vi "heating_visu OPC.vi"(7 "name":string="HT1", 9 "stop":bool, 10 "connect (T)":bool=TRUE) -> (0 "error out":errorcluster, 5 "This VI":refnum<vi>)   [LabVIEW 2019]
uses:
  ctl/Z_OnSwitch/Z_OnSwitch.xctl
  ctl/Z_ind_heating.ctl
  ctl/Z_Hswitch/Z_Hswitch.xctl
  ctl/YQ/YQ.xctl
  ctl/Y_SP/Y_SP.xctl
  ctl/Y_source.ctl
  ctl/Y_state.ctl
  ctl/Z_State.ctl
  ctl/ZM_State.ctl
  ctl/ZY_state_OPC.ctl
  ctl/ZY_state.ctl
  ctl/Z.ctl
  ctl/Y.ctl
  Inputs/Ctl/Parameter State.ctl
  Alarms/Ctl/ALR_Status.ctl
  <vilib>/OPCUA/controls/OPC UA StatusCode.ctl
  <vilib>/OPCUA/controls/Write Variant Request.ctl
  <vilib>/OPCUA/controls/NodeId.ctl
  <vilib>/OPCUA/controls/Write Status.ctl
  08a30d42-25e3-4a58-beca-1d562a75ea40.vi
  fbc51cc2-a17d-4d51-90ca-ef1d5e9adb43.vi
  3276b797-77fd-4487-96b2-8bfe15282525.vi
  81bac83f-5a8a-4521-9bb9-45d0222ee4c6.vi
  d9d9f7ca-8a59-4ad9-a7a4-c1f21956dc55.vi
  adc3267b-651c-4430-a21e-8a9f6f8285c6.vi
  45230f51-ed9d-4592-a49a-e0edfe92ddd1.vi
  Counter/Generator simplified.vi
  <vilib>/NI/AMC/Create Single Message.vi
  <vilib>/NI/AMC/Update Message Routing Info.vi
  <vilib>/NI/AMC/Read Termination Message.vi
  <vilib>/NI/AMC/Globals.vi
  <vilib>/NI/AMC/Send Message.vi
  Global stop.vi
  <vilib>/OPCUA/client/Multiple Read String.vi
  <vilib>/JDP Science/JSONtext/JSON text to Variant.vi
  <vilib>/OPCUA/client/Multiple Write Variant.vi
  Heating.lvlib
  <vilib>/OPCUA/NI OPC UA Client.lvlib
  OPC/OPC addons.lvlib
  Inputs/Inputs.lvlib
  <vilib>/NI/AMC/AMC.lvlib
  Alarms/Alarms.lvlib
panel:
  in  "Y_SP":cluster{dbl, dbl, dbl}(xcontrol)
  in  "message name":string="AI redefine"
  out "status":string
  in  "process":bool
  in  "state variables":cluster{"CurrentFile":path}
  in  "security policy":T1
  out "JSON string":string
  in  "JSON":string
  in  "Write controls":bool
  out "T stage":dbl format="%<%M:%S>t"
  in  "YQ":dbl(xcontrol)
  in  "ALRL1_reset":bool
  in  "ALRL2_reset":bool
  out "Z3 ind":T2
  out "PV":dbl(slide) caption="oC" scale=0.0..500.0 scale format="%#.1f"
  in  "Z_OnSwitch":bool(xcontrol)
  in  "Z_Hswitch":bool(xcontrol)
  in  "Y_Hswitch":bool(xcontrol)
  out "Z5 State":string
  out "Y output":dbl format="%.2f"
  # "PV"
  # "SP"
  # "Y"
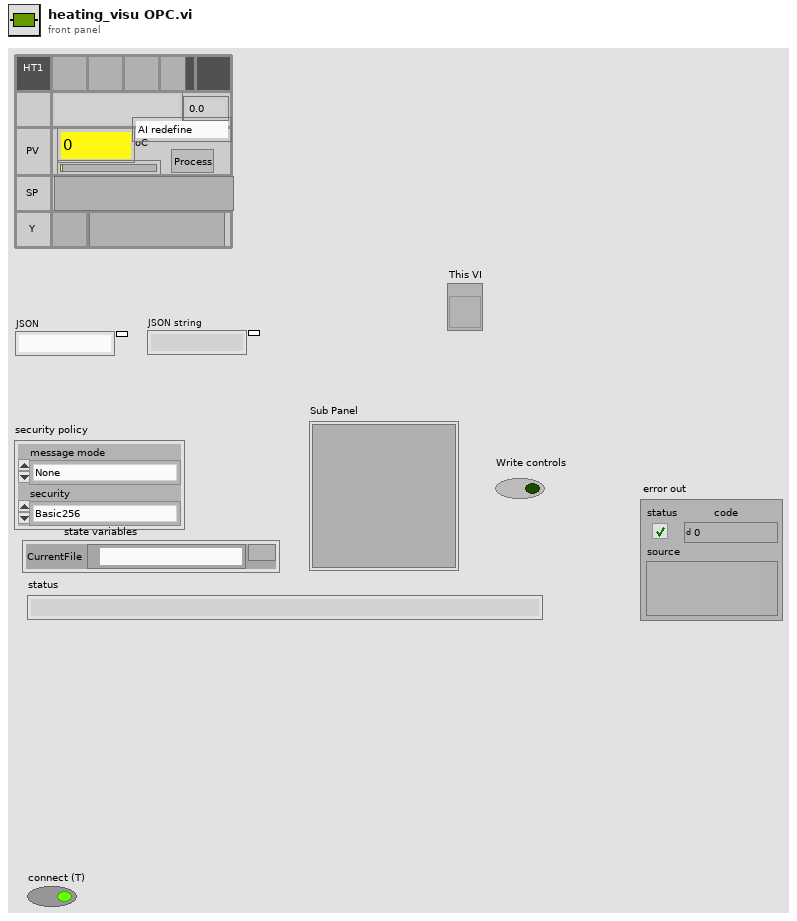
[diagram p1: front panel]
types:
  T1 = cluster{"message mode":enum16{"None", "Sign", "Sign and Encrypt"}, "security":enum16{"Basic256", "Basic128Rsa15"}}
  T2 = typedef "Heating.lvlib/Z_ind_heating.ctl" = u16
  T3 = typedef "AMC.lvlib/Message Queue.ctl" = refnum<queue>
  T4 = typedef "Write Variant Request.ctl" = cluster{"node ID":T5, "value":variant, "timestamp (current time)":timestamp, "node status":T6}
  T5 = typedef "NodeId.ctl" = string
  T6 = typedef "Write Status.ctl" = u32
  T7 = typedef "OPC UA Client Refnum.ctl" = refnum<k21>
  T8 = typedef "Subscription ID.ctl" = u32
  T9 = typedef "Heating.lvlib/Y_source.ctl" = enum8{"initialize", "local disabled", "local hand", "hand", "auto", "dist"}
  T10 = cluster{"connect":bool, "SP_Source":T9, "SP_Set":dbl, "SP":dbl}
  T11 = typedef "Heating.lvlib/Y_state.ctl" = enum8{"initialize", "alarm", "min", "stop", "hand", "auto", "max"}
  T12 = typedef "Heating.lvlib/Z_State.ctl" = enum8{"initialization", "alarm", "disabled", "not ready", "stop ready", "reserv", "switched off", "reserv2", "switched on", "check", "on min", "decrease out", "on", "increase out", "on max"}
  T13 = cluster{"connect":bool, "Z_Source":T9, "Z_State_heating":T12}
  T14 = typedef "Heating.lvlib/ZM_State.ctl" = enum8{"initialization", "stop", "start_cmd", "contactor_on_cmd", "heating", "on", "stop_cmd", "power_down", "contactor_off_cmd", "cooling", "restart_delay"}
  T15 = typedef "Heating.lvlib/ZY_state_OPC.ctl" = cluster{"Z":cluster{"Z_Source":u8, "Z_SetState":u8, "Z_State":u8, "Z_State_T":u32, "ZM_State":u8, "ZM_State_T":u32, "ALR  L1":bool, "ALR  L2":bool, "HH_run":i32}, "Y":cluster{"Y_Source":u8, "Y_SetState":u8, "SP_Set":dbl, "SP":dbl, "PV":dbl, "Y":dbl, "Y_State":cluster{"code":i32, "visible":bool, "color":u32}, "YB":bool}, "ALR_Status":cluster{"status":bool, "code":i32, "level":i32}[]}
  T16 = cluster{"Z_HSw":u32, "Z_HSetState":u32, "Y_HSw":u32, "Y_HSetState":u32, "SP":dbl, "Y_H":dbl, "Reset_ALR":bool}
  T17 = typedef "Heating.lvlib/ZY_state.ctl" = cluster{"Z":T18, "Y":T19, "ALR_Status":T21[]}
  T18 = typedef "Heating.lvlib/Z.ctl" = cluster{"Z_Source":T9, "Z_SetState":T12, "Z_State":T12, "Z_State_T":u32, "ZM_State":T14, "ZM_State_T":u32, "ALR  L1":bool, "ALR  L2":bool, "HH_run":i32}
  T19 = typedef "Heating.lvlib/Y.ctl" = cluster{"Y_Source":T9, "Y_SetState":T11, "SP_Set":dbl, "SP":dbl, "PV":dbl, "Y":dbl, "Y_State":T20, "YB":bool}
  T20 = typedef "Inputs.lvlib/Parameter State.ctl" = cluster{"code":i32, "visible":bool, "color":u32, "source":string}
  T21 = typedef "Alarms.lvlib/ALR_Status.ctl" = cluster{"status":bool, "code":i32, "level":i32, "source":string}
  T22 = typedef "OPC UA StatusCode.ctl" = u32
  T23 = enum32{"Invalid Status", "Unconnected", "Active", "Idle", "Error", "Connecting"}
  T24 = cluster{"node ID":T5, "value ":string, "timestamp":timestamp, "status":T22}[]
  T25 = typedef "LVDataSocketStatusTypeDef.ctl" = cluster{"Code":enum32{"Invalid Status", "Unconnected", "Active", "Idle", "Error", "Connecting"}, "Text":string}
  T26 = cluster{"node ID":T5, "value ":string, "timestamp":timestamp, "status":T22}
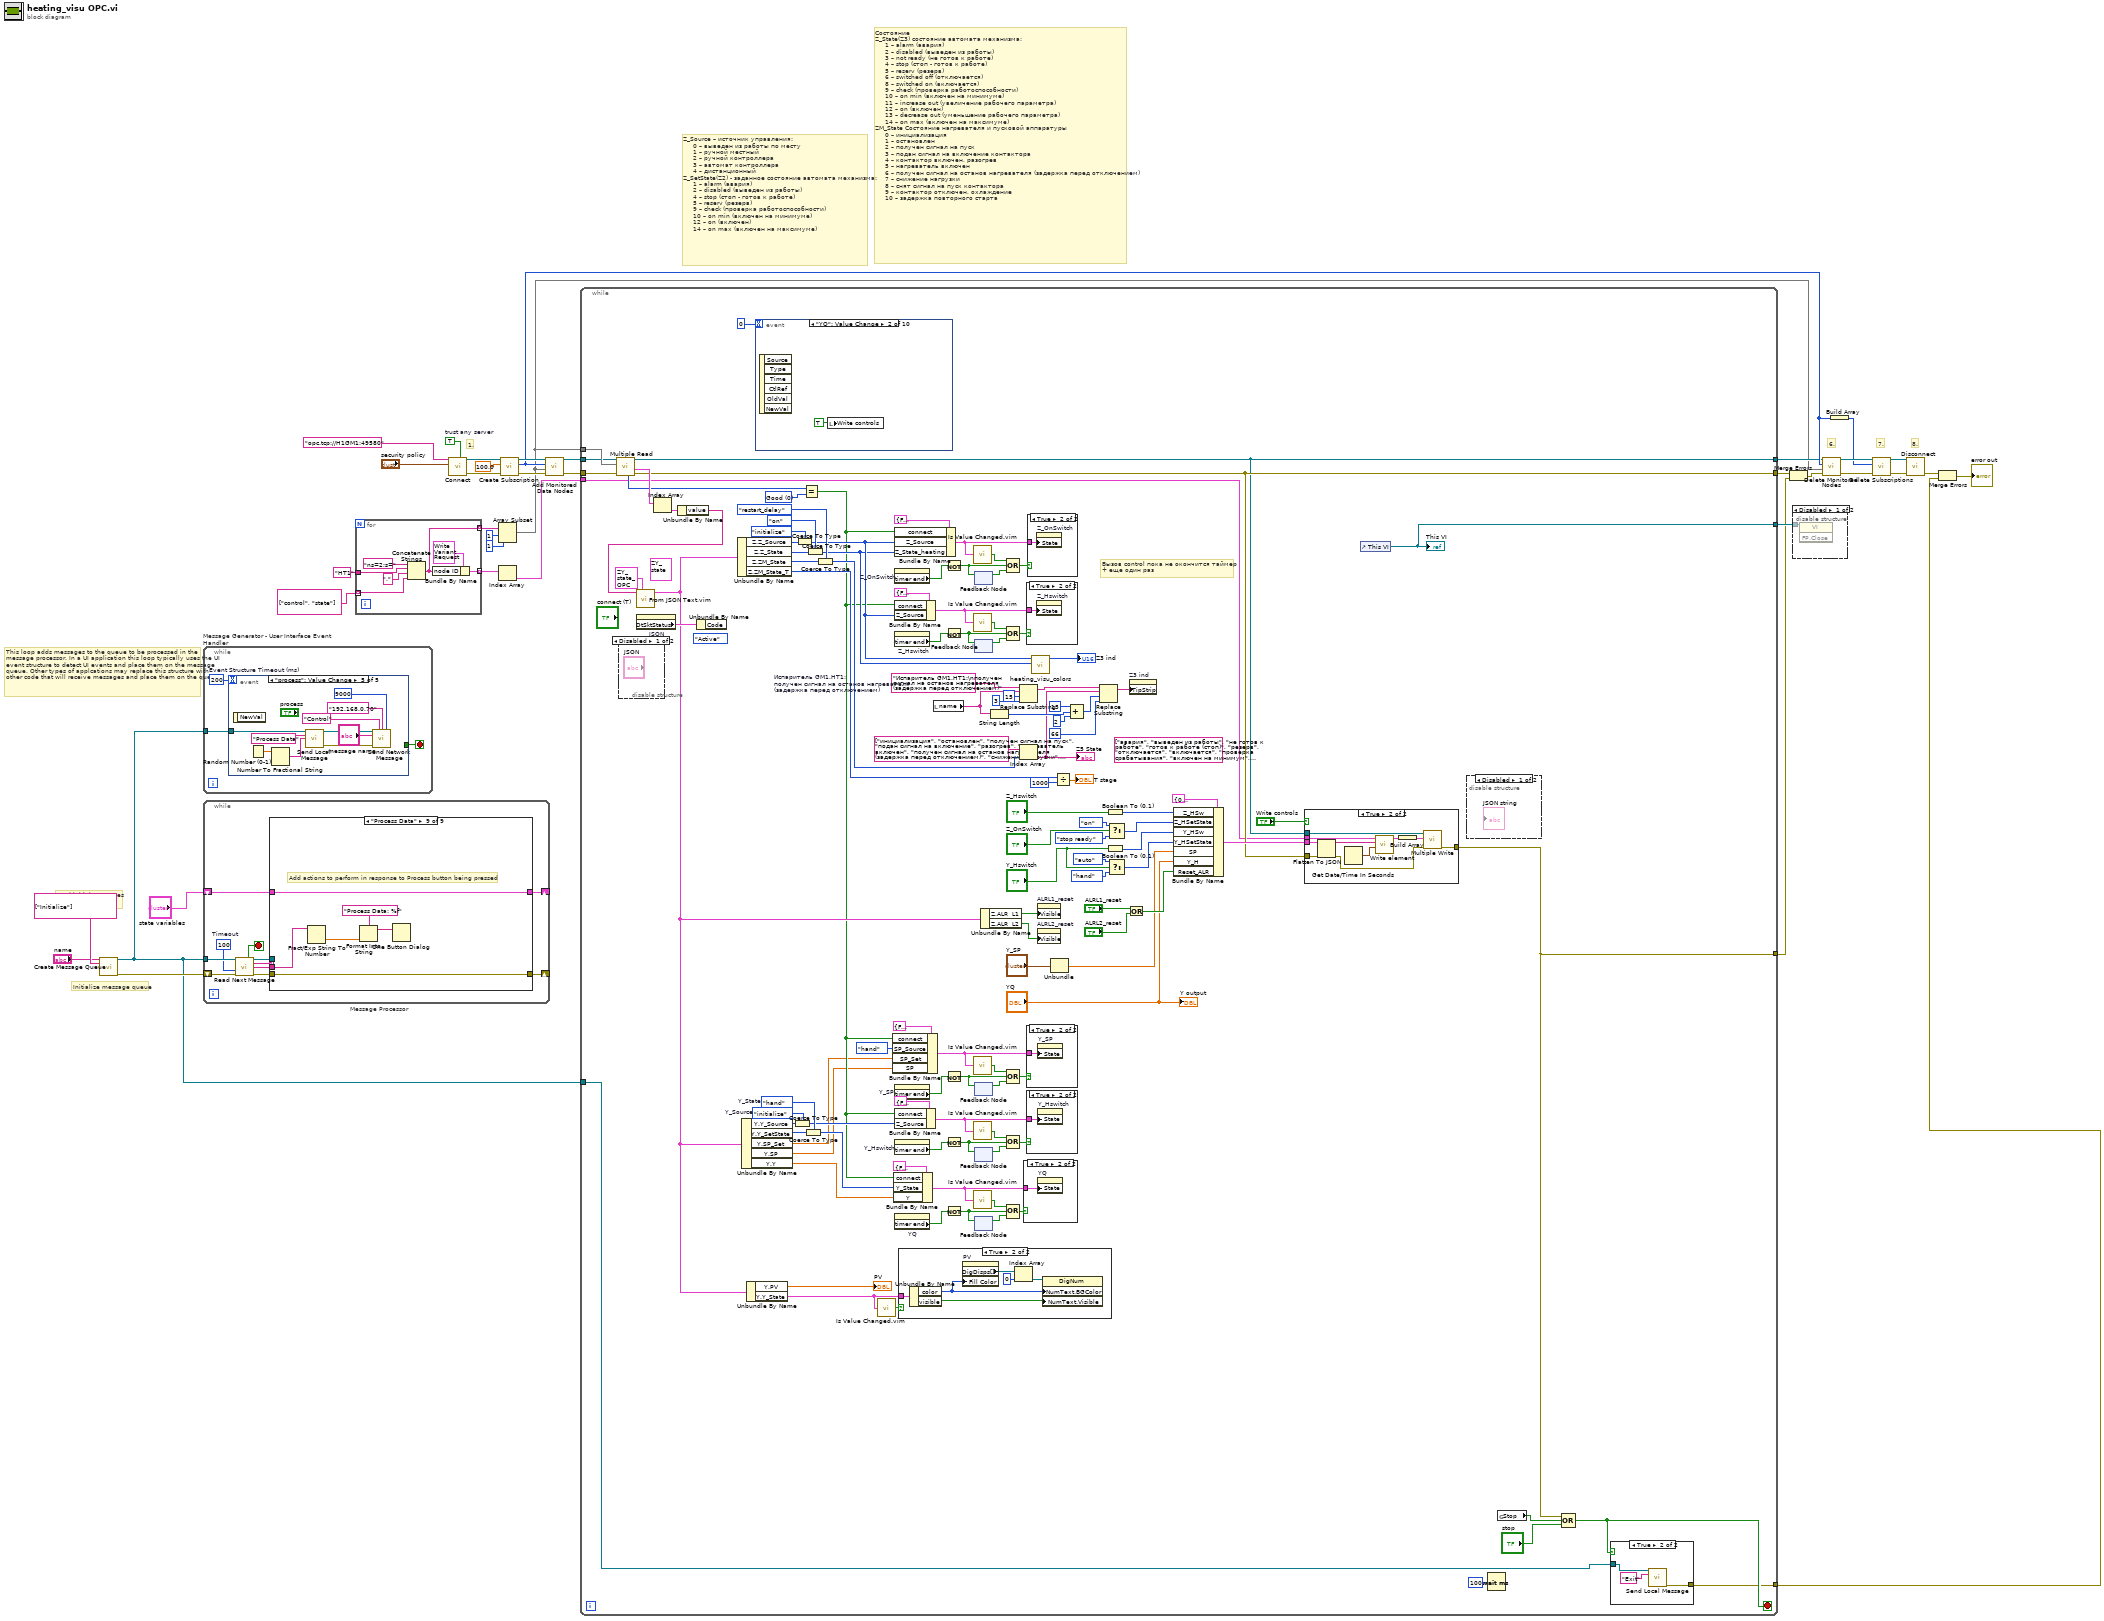
[diagram p0: block diagram]
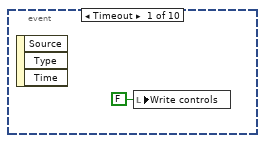
[diagram p9: hidden frame]
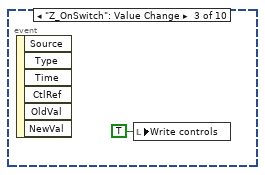
[diagram p10: hidden frame]
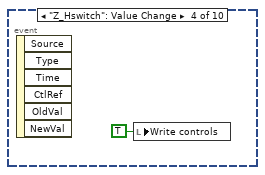
[diagram p11: hidden frame]
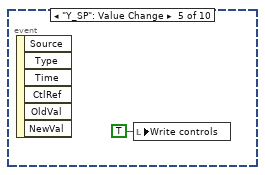
[diagram p12: hidden frame]
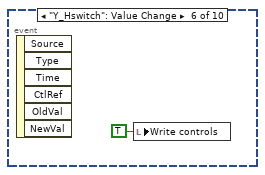
[diagram p13: hidden frame]
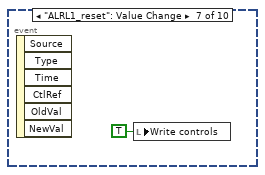
[diagram p14: hidden frame]
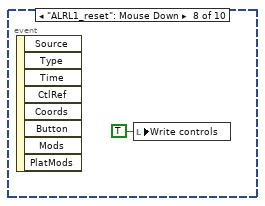
[diagram p15: hidden frame]
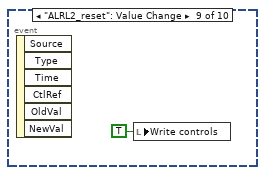
[diagram p16: hidden frame]
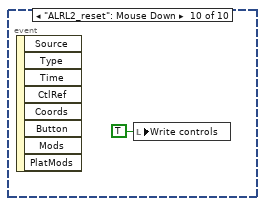
[diagram p17: hidden frame]
diagram:
  w30 = TRUE  # trust any server
  # "This loop adds messages to the queue to be processed in the message processor. In a UI application this loop typically uses the UI event structure to detect UI events and place them on the message queue. Other types of applcations may replace this structure with other code that will receive messages and place them on the queue."
  # "Initialize message queue"
  # "Load initial messages\non the queue"
  # "7."
  # "8."
  # "6."
  # "1."
  # "Состояние\nZ_State(Z3) состояние автомата механизма:\n     1 – alarm (авария)\n     2 – disabled (выведен из работы)\n     3 – not ready (не готов к работе)\n     4 – stop (стоп - готов к работе)\n     5 – reserv (резерв)\n     6 – switched off (отключается)\n     8 – switched on (включается)\n     9 – check (проверка работоспособности)\n     10 – on min (включен на минимуме)\n     11 – increase out (увеличение рабочего параметра)\n     12 – on (включен)\n     13 – decrease out (уменьшение рабочего параметра)\n     14 – on max (включен на максимуме)\nZM_State Состояние нагревателя и пусковой аппаратуры\n     0 – инициализация\n     1 – остановлен\n     2 – получен сигнал на пуск\n     3 – подан сигнал на включение контактора\n     4 – контактор включен, разогрев\n     5 – нагреватель включен\n     6 – получен сигнал на останов нагревателя (задержка перед отключением)\n     7 – снижение нагрузки\n     8 – снят сигнал на пуск контактора\n     9 – контактор отключен, охлаждение\n     10 – задержка повторного старта"
  # "Z_Source – источник управления:\n     0 – выведен из работы по месту\n     1 – ручной местный\n     2 – ручной контроллера\n     3 – автомат контроллера\n     4 – дистанционный\nZ_SetState(Z2) - заданное состояние автомата механизма:\n     1 – alarm (авария)\n     2 – disabled (выведен из работы)\n     4 – stop (стоп - готов к работе)\n     5 – reserv (резерв)\n     9 – check (проверка работоспособности)\n     10 – on min (включен на минимуме)\n     12 – on (включен)\n     14 – on max (включен на максимуме)"
  n1 = call <vilib>:"Create Message Queue.vi"("message queue name"="name", "initial message names"=string[] ["Initialize"]) -> ("message queue out"=w5:T3, "error out"=w7:errorcluster)  [unwired: 12 in]
  n2 = while "Message Generator - User Interface Event Handler" {
    tunnel: w5 -> [w38]
    stop <- w39 stop-if-true
    w40 = 200  # Event Structure Timeout (ms)
    n3 = event shown="[4] \"process\": Value Change" {
      selector: _ -> [_ _ _ _ _]
      dyn-events: _ -> [_ _ _ _ _]
      timeout: w40 -> [_ _ _ _ _]
      tunnel: [w41 w46 TRUE ("Discard?") _ _] -> w39
      tunnel: w38 -> [w42 w44 w47 w50 w61]
      event Timeout {
        # "Exit UI event handler loop if message queue\nis destroyed in the message processor"
        n4 = event-data() -> ()  [unwired: 2 out]
        n5 = call <vilib>:"Check Message Queue Status.vi"("message queue in"=w42) -> ("error out"=w43:errorcluster)  [unwired: 10 in, 4 out]
        n6 = Unbundle By Name(w43) -> ("status"=w41:bool)
        n7 = local write "stop"(w41) -> ()
      }
      event Panel Close? {
        w46 = TRUE ("Discard?")
        # "Intercepts the upper right close panel\noperation to allow a smooth shutdown\nas opposed to immediately killing the app."
        n8 = event-data() -> ()  [unwired: 2 out]
        n9 = call <vilib>:"Send Local Message.vi"("message queue in"=w44, "message name"="Exit") -> ()  [unwired: 11 in, 3 out]
        n10 = event-data("Discard?"=w46) -> ()  [unwired: 1 in, 1 out]
      }
      event "stop": Value Change {
        # "Exit the application\n>> Stop this message generator loop"
        n11 = event-data() -> ()  [unwired: 7 out]
        n12 = call <vilib>:"Send Local Message.vi"("message queue in"=w47, "message name"="Exit") -> ()  [unwired: 11 in, 3 out]
      }
      event Menu Selection (User) {
        # "Add run-time menu items to the message\nqueue. The message handler case names must match the menu ItemTag names."
        n13 = event-data() -> ("ItemTag"=w51:string)  [unwired: 1 out]
        n14 = call <vilib>:"Send Local Message.vi"("message queue in"=w50, "message name"=w51) -> ()  [unwired: 11 in, 3 out]
      }
      event "process": Value Change {
        n15 = event-data() -> ()  [unwired: 2 out]
        n16 = Random Number (0-1)() -> (number: 0 to 1=w58:dbl)
        n17 = Number To Fractional String(number=w58) -> (F-format string=w59:string)  [unwired: 3 out]
        n18 = call <vilib>:"Send Local Message.vi"("message queue in"=w61, "message name"="Process Data", "message value"=w59) -> ("message queue out"=w57:T3, "error out"=w53:errorcluster)  [unwired: 10 in, 1 out]
        n19 = call <vilib>:"Send Network Message.vi"("message queue in"=w57, "receiver process"="Control", "receiver host"="192.168.0.70", "receiver port (0)"=u16 9000, "message name"="message name", "error in"=w53) -> ()  [unwired: 7 in, 3 out]
      }
    }
  }
  n20 = while "Message Processor" {
    shift-left: w7 -> [w66]
    shift-right: [w70] -> _
    tunnel: w5 -> [w67]
    shift-left: "state variables" -> [w72]
    shift-right: [w71] -> _
    stop <- w69 stop-if-true
    w62 = 100  # Timeout
    n21 = call <vilib>:"Read Next Message.vi"("message queue in"=w67, "timeout (1 ms)"=w62, "error in"=w66) -> ("exit process?"=w69:bool, "message queue out"=w68:T3, "message name"=w64:string, "message value"=w63:string, "error out"=w65:errorcluster)  [unwired: 5 in, 3 out]
    n22 = case shown="\"Process Data\"" w64 {
      selector: w64 -> [_ _ w84 _ _ _ _ _ _]
      tunnel: [w74 w81 w86 w91 w93 w95 w100 w102 w107] -> w71
      tunnel: w72 -> [w74 w81 w86 w91 w93 w95 w100 w102 w107]
      tunnel: w68 -> [_ _ _ w89 _ _ w97 _ _]
      tunnel: w65 -> [w73 w80 w85 w87 w92 w94 w98 w101 w108]
      tunnel: [w73 w80 w85 errorcluster {"status"=FALSE, "code"=0, "source"=""} ("error out") w92 w94 w96 w101 w108] -> w70
      tunnel: w63 -> [_ _ _ _ _ _ _ _ w106]
      frame "---------- Framework Operations ----------" {
        # "Dummy case to add a seperator in the Case Structure menu"
      }
      frame "", "Idle" {
        # "Update the front panel"
        # "Idle Case - this case is called after a Timeout on the Get Next Message from Queue VI, if no new messages are present on the queue. This case can be used for housekeeping tasks such as updating the UI."
        n23 = Get Date/Time String(want seconds? (F)=TRUE) -> (date string=w79:string, time string=w78:string)  [unwired: 2 out]
        n24 = Concatenate Strings(w79, " " ("string"), w78) -> (→"status":string)
      }
      frame "Missing Message Handler", Default {
        # "Call this case if a message is received that is not handled \nby any other case. Typically this is a programming error\nas a result of a typo or unhandled message/missing message handler."
        n25 = Format Into String(format string="DevError: Missing message handler for '%s\" message." ("message"), w84) -> (resulting string=w82:string)  [unwired: 2 in, 1 out]
        n26 = One Button Dialog(message=w82) -> ()  [unwired: 2 out]
      }
      frame "Error" {
        # "Proceed to Exit - Remove this if it is\nnot appropriate for the General Error case"
        # "General Error Case - this case is called if an error is passed using the error cluster below. Typically most new errors should be handed in each individual case and not passed in the rror cluster. If necessary a custom error handler case should be added and called from other cases."
        n27 = call <vilib>:"Simple Error Handler.vi"("error in (no error)"=w87) -> ()  [unwired: 1 in, 8 out]
        n28 = call <vilib>:"Send Local Message.vi"("message queue in"=w89, "message name"="Exit") -> ()  [unwired: 11 in, 3 out]
      }
      frame "---------- Generic Operations ----------" {
        # "Dummy case to add a seperator in the Case Structure menu"
      }
      frame "Initialize" {
        # "Initialize the state variables and user interface"
      }
      frame "Exit" {
        # "Destroy message queue >> this will halt the UI event handler loop"
        # "Stop the VI\n>> Perform any cleanup tasks in this message case.\n>> Clear display before closing."
        n29 = call <vilib>:"Destroy Message Queue.vi"("message queue in"=w97, "error in"=w98) -> ("error out"=w96:errorcluster)  [unwired: 11 in, 2 out]
        n30 = local write "status"("" ("Status")) -> ()
      }
      frame "---------- Application Operations ----------" {
        # "Dummy case to add a seperator in the Case Structure menu"
      }
      frame "Process Data" {
        # "Add actions to perform in response to Process button being pressed"
        n31 = Fract/Exp String To Number(string=w106) -> (number=w105:dbl)  [unwired: 4 out]
        n32 = Format Into String(format string="Process Data: %f" ("message"), w105) -> (resulting string=w103:string)  [unwired: 2 in, 1 out]
        n33 = One Button Dialog(message=w103) -> ()  [unwired: 2 out]
      }
    }
  }
  n34 = for {
    tunnel: string[] ["control", "state"] -> [w109] mode=indexing
    tunnel: "HT1" ("Folder Name") -> [w115]
    tunnel: [w112] -> w19 mode=indexing
    tunnel: [w111] -> w15 mode=indexing
    n35 = Concatenate Strings("ns=2;s=" ("string"), w115, "." ("string"), w109) -> (w112:string)
    n36 = Bundle By Name(cluster=T4 {"node ID"="", "value"=variant, "timestamp (current time)"=timestamp(0 s since 1904-01-01), "node status"=0} ("request"), "node ID"=w112) -> (w111:T4)
  }
  n37 = call <vilib>:"Connect.vi"("trust any server (F)"=w30, "security policy"="security policy", "server endpoint URL"="opc.tcp://H1GM1:49580" ("server endpoint URL 2")) -> ("error out"=w33:errorcluster, "OPC UA client refnum out"=w34:T7)  [unwired: 6 in, 1 out]
  n38 = Array Subset(array=w19, index=1, length=1) -> (w9:string[])
  n39 = Index Array(array=w15) -> (element=w13:T4)  [unwired: 1 in]
  n40 = call <vilib>:"Create Subscription.vi"("error in (no error)"=w33, "publishing interval (1000 ms)"=100.0 ("update rate (1000 ms)"), "OPC UA client refnum in"=w34) -> ("error out"=w35:errorcluster, "subscription ID out"=w23:T8, "OPC UA client refnum out"=w36:T7)  [unwired: 4 in, 2 out]
  n41 = call <vilib>:"Add Monitored Data Nodes.vi"("error in (no error)"=w35, "node IDs"=w9, "subscription ID in"=w23, "OPC UA client refnum in"=w36) -> ("error out"=w16:errorcluster, "OPC UA client refnum out"=w17:T7)  [unwired: 4 in, 2 out]
  n42 = while {
    tunnel: [w198] -> w37
    tunnel: w17 -> [w187]
    tunnel: w16 -> [w194]
    tunnel: w13 -> [w186]
    tunnel: [w185] -> w12
    tunnel: [w187] -> w11
    tunnel: [w189] -> w10
    tunnel: w9 -> [w193]
    tunnel: w5 -> [w183]
    tunnel: [w182] -> w3
    stop <- w184 stop-if-true
    w170 = Y_state."hand"  # Y_State
    w171 = Y_source."initialize"  # Y_Source
    (unwired) T17 {"Z"={"Z_Source"=enum."initialize", "Z_SetState"=enum."initialization", "Z_State"=enum."initialization", "Z_State_T"=0, "ZM_State"=enum."initialization", "ZM_State_T"=0, "ALR  L1"=FALSE, "ALR  L2"=FALSE, "HH_run"=0}, "Y"={"Y_Source"=enum."initialize", "Y_SetState"=enum."initialize", "SP_Set"=0.0, "SP"=0.0, "PV"=0.0, "Y"=0.0, "Y_State"={"code"=0, "visible"=FALSE, "color"=0, "source"=""}, "YB"=FALSE}, "ALR_Status"=[]} ("HT1_state")
    w191 = T22 0 items=["Good"=0, "Good_SubscriptionTransferred"=2949120, "Good_CompletesAsynchronously"=3014656, "Good_Overload"=3080192, "Good_Clamped"=3145728, "Good_LocalOverride"=9830400, "Good_EntryInserted"=10616832, "Good_EntryReplaced"=10682368, "Good_NoData"=10813440, "Good_MoreData"=10878976, "Good_CommunicationEvent"=10944512, "Good_ShutdownEvent"=11010048, "Good_CallAgain"=11075584, "Good_NonCriticalTimeout"=11141120, "Good_ResultsMayBeIncomplete"=12189696, "Good_DataIgnored"=14221312, "Uncertain"=1073741824, "Uncertain_ReferenceOutOfServer"=1080819712, "Uncertain_NoCommunicationLastUsableValue"=1083113472, "Uncertain_LastUsableValue"=1083179008, "Uncertain_SubstituteValue"=1083244544, "Uncertain_InitialValue"=1083310080, "Uncertain_SensorNotAccurate"=1083375616, "Uncertain_EngineeringUnitsExceeded"=1083441152, "Uncertain_SubNormal"=1083506688, "Uncertain_DataSubNormal"=1084489728, "Uncertain_ReferenceNotDeleted"=1086062592, "Uncertain_NotAllNodesAvailable"=1086324736, "Bad"=2147483648, "Bad_UnexpectedError"=2147549184, "Bad_InternalError"=2147614720, "Bad_OutOfMemory"=2147680256, "Bad_ResourceUnavailable"=2147745792, "Bad_CommunicationError"=2147811328, "Bad_EncodingError"=2147876864, "Bad_DecodingError"=2147942400, "Bad_EncodingLimitsExceeded"=2148007936, "Bad_UnknownResponse"=2148073472, "Bad_Timeout"=2148139008, "Bad_ServiceUnsupported"=2148204544, "Bad_Shutdown"=2148270080, "Bad_ServerNotConnected"=2148335616, "Bad_ServerHalted"=2148401152, "Bad_NothingToDo"=2148466688, "Bad_TooManyOperations"=2148532224, "Bad_DataTypeIdUnknown"=2148597760, "Bad_CertificateInvalid"=2148663296, "Bad_SecurityChecksFailed"=2148728832, "Bad_CertificateTimeInvalid"=2148794368, "Bad_CertificateIssuerTimeInvalid"=2148859904, "Bad_CertificateHostNameInvalid"=2148925440, "Bad_CertificateUriInvalid"=2148990976, "Bad_CertificateUseNotAllowed"=2149056512, "Bad_CertificateIssuerUseNotAllowed"=2149122048, "Bad_CertificateUntrusted"=2149187584, "Bad_CertificateRevocationUnknown"=2149253120, "Bad_CertificateIssuerRevocationUnknown"=2149318656, "Bad_CertificateRevoked"=2149384192, "Bad_CertificateIssuerRevoked"=2149449728, "Bad_UserAccessDenied"=2149515264, "Bad_IdentityTokenInvalid"=2149580800, "Bad_IdentityTokenRejected"=2149646336, "Bad_SecureChannelIdInvalid"=2149711872, "Bad_InvalidTimestamp"=2149777408, "Bad_NonceInvalid"=2149842944, "Bad_SessionIdInvalid"=2149908480, "Bad_SessionClosed"=2149974016, "Bad_SessionNotActivated"=2150039552, "Bad_SubscriptionIdInvalid"=2150105088, "Bad_RequestHeaderInvalid"=2150236160, "Bad_TimestampsToReturnInvalid"=2150301696, "Bad_RequestCancelledByClient"=2150367232, "Bad_NoCommunication"=2150694912, "Bad_WaitingForInitialData"=2150760448, "Bad_NodeIdInvalid"=2150825984, "Bad_NodeIdUnknown"=2150891520, "Bad_AttributeIdInvalid"=2150957056, "Bad_IndexRangeInvalid"=2151022592, "Bad_IndexRangeNoData"=2151088128, "Bad_DataEncodingInvalid"=2151153664, "Bad_DataEncodingUnsupported"=2151219200, "Bad_NotReadable"=2151284736, "Bad_NotWritable"=2151350272, "Bad_OutOfRange"=2151415808, "Bad_NotSupported"=2151481344, "Bad_NotFound"=2151546880, "Bad_ObjectDeleted"=2151612416, "Bad_NotImplemented"=2151677952, "Bad_MonitoringModeInvalid"=2151743488, "Bad_MonitoredItemIdInvalid"=2151809024, "Bad_MonitoredItemFilterInvalid"=2151874560, "Bad_MonitoredItemFilterUnsupported"=2151940096, "Bad_FilterNotAllowed"=2152005632, "Bad_StructureMissing"=2152071168, "Bad_EventFilterInvalid"=2152136704, "Bad_ContentFilterInvalid"=2152202240, "Bad_FilterOperandInvalid"=2152267776, "Bad_ContinuationPointInvalid"=2152333312, "Bad_NoContinuationPoints"=2152398848, "Bad_ReferenceTypeIdInvalid"=2152464384, "Bad_BrowseDirectionInvalid"=2152529920, "Bad_NodeNotInView"=2152595456, "Bad_ServerUriInvalid"=2152660992, "Bad_ServerNameMissing"=2152726528, "Bad_DiscoveryUrlMissing"=2152792064, "Bad_SempahoreFileMissing"=2152857600, "Bad_RequestTypeInvalid"=2152923136, "Bad_SecurityModeRejected"=2152988672, "Bad_SecurityPolicyRejected"=2153054208, "Bad_TooManySessions"=2153119744, "Bad_UserSignatureInvalid"=2153185280, "Bad_ApplicationSignatureInvalid"=2153250816, "Bad_NoValidCertificates"=2153316352, "Bad_RequestCancelledByRequest"=2153381888, "Bad_ParentNodeIdInvalid"=2153447424, "Bad_ReferenceNotAllowed"=2153512960, "Bad_NodeIdRejected"=2153578496, "Bad_NodeIdExists"=2153644032, "Bad_NodeClassInvalid"=2153709568, "Bad_BrowseNameInvalid"=2153775104, "Bad_BrowseNameDuplicated"=2153840640, "Bad_NodeAttributesInvalid"=2153906176, "Bad_TypeDefinitionInvalid"=2153971712, "Bad_SourceNodeIdInvalid"=2154037248, "Bad_TargetNodeIdInvalid"=2154102784, "Bad_DuplicateReferenceNotAllowed"=2154168320, "Bad_InvalidSelfReference"=2154233856, "Bad_ReferenceLocalOnly"=2154299392, "Bad_NoDeleteRights"=2154364928, "Bad_ServerIndexInvalid"=2154430464, "Bad_ViewIdUnknown"=2154496000, "Bad_TooManyMatches"=2154627072, "Bad_QueryTooComplex"=2154692608, "Bad_NoMatch"=2154758144, "Bad_MaxAgeInvalid"=2154823680, "Bad_HistoryOperationInvalid"=2154889216, "Bad_HistoryOperationUnsupported"=2154954752, "Bad_WriteNotSupported"=2155020288, "Bad_TypeMismatch"=2155085824, "Bad_MethodInvalid"=2155151360, "Bad_ArgumentsMissing"=2155216896, "Bad_TooManySubscriptions"=2155282432, "Bad_TooManyPublishRequests"=2155347968, "Bad_NoSubscription"=2155413504, "Bad_SequenceNumberUnknown"=2155479040, "Bad_MessageNotAvailable"=2155544576, "Bad_InsufficientClientProfile"=2155610112, "Bad_TcpServerTooBusy"=2155675648, "Bad_TcpMessageTypeInvalid"=2155741184, "Bad_TcpSecureChannelUnknown"=2155806720, "Bad_TcpMessageTooLarge"=2155872256, "Bad_TcpNotEnoughResources"=2155937792, "Bad_TcpInternalError"=2156003328, "Bad_TcpEndpointUrlInvalid"=2156068864, "Bad_RequestInterrupted"=2156134400, "Bad_RequestTimeout"=2156199936, "Bad_SecureChannelClosed"=2156265472, "Bad_SecureChannelTokenUnknown"=2156331008, "Bad_SequenceNumberInvalid"=2156396544, "Bad_ConfigurationError"=2156462080, "Bad_NotConnected"=2156527616, "Bad_DeviceFailure"=2156593152, "Bad_SensorFailure"=2156658688, "Bad_OutOfService"=2156724224, "Bad_DeadbandFilterInvalid"=2156789760, "Bad_RefreshInProgress"=2157379584, "Bad_ConditionAlreadyDisabled"=2157445120, "Bad_ConditionDisabled"=2157510656, "Bad_EventIdUnknown"=2157576192, "Bad_NoData"=2157641728, "Bad_DataLost"=2157772800, "Bad_DataUnavailable"=2157838336, "Bad_EntryExists"=2157903872, "Bad_NoEntryExists"=2157969408, "Bad_TimestampNotSupported"=2158034944, "Bad_InvalidArgument"=2158690304, "Bad_ConnectionRejected"=2158755840, "Bad_Disconnect"=2158821376, "Bad_ConnectionClosed"=2158886912, "Bad_InvalidState"=2158952448, "Bad_EndOfStream"=2159017984, "Bad_NoDataAvailable"=2159083520, "Bad_WaitingForResponse"=2159149056, "Bad_OperationAbandoned"=2159214592, "Bad_ExpectedStreamToBlock"=2159280128, "Bad_WouldBlock"=2159345664, "Bad_SyntaxError"=2159411200, "Bad_MaxConnectionsReached"=2159476736, "Bad_RequestTooLarge"=2159542272, "Bad_ResponseTooLarge"=2159607808, "Bad_EventNotAcknowledgeable"=2159738880, "Bad_InvalidTimestampArgument"=2159869952, "Bad_ProtocolVersionUnsupported"=2159935488, "Bad_StateNotActive"=2160001024, "Bad_FilterOperatorInvalid"=2160132096, "Bad_FilterOperatorUnsupported"=2160197632, "Bad_FilterOperandCountMismatch"=2160263168, "Bad_FilterElementInvalid"=2160328704, "Bad_FilterLiteralInvalid"=2160394240, "Bad_IdentityChangeNotSupported"=2160459776, "Bad_NotTypeDefinition"=2160590848, "Bad_ViewTimestampInvalid"=2160656384, "Bad_ViewParameterMismatch"=2160721920, "Bad_ViewVersionInvalid"=2160787456, "Bad_ConditionAlreadyEnabled"=2160852992, "Bad_DialogNotActive"=2160918528, "Bad_DialogResponseInvalid"=2160984064, "Bad_ConditionBranchAlreadyAcked"=2161049600, "Bad_ConditionBranchAlreadyConfirmed"=2161115136, "Bad_ConditionAlreadyShelved"=2161180672, "Bad_ConditionNotShelved"=2161246208, "Bad_ShelvingTimeOutOfRange"=2161311744, "Bad_AggregateListMismatch"=2161377280, "Bad_AggregateNotSupported"=2161442816, "Bad_AggregateInvalidInputs"=2161508352, "Bad_BoundNotFound"=2161573888, "Bad_BoundNotSupported"=2161639424, "Bad_AggregateConfigurationRejected"=2161770496, "Bad_TooManyMonitoredItems"=2161836032] ("y")
    (unwired) T23."Active" ("Code")
    (unwired) string[] ["авария", "выведен из работы", "не готов к работе", "готов к работе (стоп)", "резерв", "отключается", "включается", "проверка срабатывания", "включен на минимум", "увеличение произв", "включен", "уменьшение произв", "включен на максимум"]
    w231 = "Испаритель GM1.HT1:\nполучен сигнал на останов нагревателя (задержка перед отключением)"  # Испаритель GM1.HT1: получен сигнал на останов нагревателя (задержка перед отключением)
    # "Вызов control пока не окончится таймер\n+ еще один раз"
    n43 = call-poly <vilib>:"Multiple Read.vi"("error in (no error)"=w194, "node IDs"=w193, "OPC UA client refnum in"=w187) -> ("error out"=w189:errorcluster, "results"=w196:T24, "service status"=w192:T22)  [unwired: 5 in, 1 out]
    n44 = disable-structure shown="Disabled" {
      frame Disabled {
      }
      frame Enabled {
      }
    }
    n45 = property on="JSON" class="Str"() -> ("DtSktStatus"=w199:T25)  [unwired: 2 in, 2 out]
    n46 = Index Array(array=w196) -> (element=w195:T26)  [unwired: 1 in]
    n47 = Unbundle By Name(w195) -> ("value"=w188:string)
    n48 = call "From JSON Text.vim"("Data Type and Default Value"=T15 {"Z"={"Z_Source"=0, "Z_SetState"=0, "Z_State"=0, "Z_State_T"=0, "ZM_State"=0, "ZM_State_T"=0, "ALR  L1"=FALSE, "ALR  L2"=FALSE, "HH_run"=0}, "Y"={"Y_Source"=0, "Y_SetState"=0, "SP_Set"=0.0, "SP"=0.0, "PV"=0.0, "Y"=0.0, "Y_State"={"code"=0, "visible"=FALSE, "color"=0}, "YB"=FALSE}, "ALR_Status"=[]} ("ZY_State"), "JSON"=w188) -> ("Data out"=w134:T15)  [unwired: 8 in, 1 out]
    n49 = Unbundle By Name(w199) -> ()  [unwired: 1 out]
    n50 = Unbundle By Name(w134) -> ("Z.Z_Source"=w177:u8, "Z.Z_State"=w211:u8, "Z.ZM_State"=w206:u8, "Z.ZM_State_T"=w213:u32)
    n51 = Unbundle By Name(w134) -> ("Y.Y_Source"=w176:u8, "Y.Y_SetState"=w212:u8, "Y.SP_Set"=w120:dbl, "Y.SP"=w119:dbl, "Y.Y"=w130:dbl)
    n52 = Unbundle By Name(w134) -> ("Y.PV"=→"PV":dbl, "Y.Y_State"=w132:cluster{"code":i32, "visible":bool, "color":u32})
    n53 = event shown="[1] \"YQ\": Value Change" {
      selector: _ -> [_ _ _ _ _ _ _ _ _ _]
      dyn-events: _ -> [_ _ _ _ _ _ _ _ _ _]
      timeout: 0 -> [_ _ _ _ _ _ _ _ _ _]
      event Timeout {
        n54 = event-data() -> ()  [unwired: 1 in, 3 out]
        n55 = local write "Write controls"(FALSE ("manual_reset")) -> ()
      }
      event "YQ": Value Change {
        n56 = event-data() -> ()  [unwired: 1 in, 6 out]
        n57 = local write "Write controls"(TRUE ("manual_reset")) -> ()
      }
      event "Z_OnSwitch": Value Change {
        n58 = event-data() -> ()  [unwired: 1 in, 6 out]
        n59 = local write "Write controls"(TRUE ("manual_reset")) -> ()
      }
      event "Z_Hswitch": Value Change {
        n60 = event-data() -> ()  [unwired: 1 in, 6 out]
        n61 = local write "Write controls"(TRUE ("manual_reset")) -> ()
      }
      event "Y_SP": Value Change {
        n62 = event-data() -> ()  [unwired: 1 in, 6 out]
        n63 = local write "Write controls"(TRUE ("manual_reset")) -> ()
      }
      event "Y_Hswitch": Value Change {
        n64 = event-data() -> ()  [unwired: 1 in, 6 out]
        n65 = local write "Write controls"(TRUE ("manual_reset")) -> ()
      }
      event "ALRL1_reset": Value Change {
        n66 = event-data() -> ()  [unwired: 1 in, 6 out]
        n67 = local write "Write controls"(TRUE ("manual_reset")) -> ()
      }
      event "ALRL1_reset": Mouse Down {
        n68 = event-data() -> ()  [unwired: 1 in, 8 out]
        n69 = local write "Write controls"(TRUE ("manual_reset")) -> ()
      }
      event "ALRL2_reset": Value Change {
        n70 = event-data() -> ()  [unwired: 1 in, 6 out]
        n71 = local write "Write controls"(TRUE ("manual_reset")) -> ()
      }
      event "ALRL2_reset": Mouse Down {
        n72 = event-data() -> ()  [unwired: 1 in, 8 out]
        n73 = local write "Write controls"(TRUE ("manual_reset")) -> ()
      }
    }
    n74 = Coerce To Type(0:w176, 1:w171) -> (2:w131:T9)
    n75 = Coerce To Type(0:w177, 1:Y_source."initialize" ("Y_Source")) -> (2:w161:T9)
    n76 = Equal?(x=w192, y=w191) -> (x = y?=w121:bool)
    n77 = Coerce To Type(0:w212, 1:w170) -> (2:w129:T11)
    n78 = Coerce To Type(0:w211, 1:Z_State."on" ("Z_State_heating")) -> (2:w160:T12)
    n79 = Coerce To Type(0:w206, 1:ZM_State."restart_delay" ("ZM_State_heating")) -> (2:w173:T14)
    n80 = call "Is Value Changed.vim"("value"=w132) -> ("changed or first call?"=w156:bool)
    n81 = Bundle By Name(cluster=T10 {"connect"=FALSE, "SP_Source"=enum."initialize", "SP_Set"=0.0, "SP"=0.0} ("source"), "connect"=w121, "SP_Source"=Y_source."hand", "SP_Set"=w120, "SP"=w119) -> (w128:T10)
    n82 = Bundle By Name(cluster=cluster{"connect":bool, "Y_State":T11, "Y":dbl} {"connect"=FALSE, "Y_State"=enum."initialize", "Y"=0.0} ("source"), "connect"=w121, "Y_State"=w129, "Y"=w130) -> (w142:cluster{"connect":bool, "Y_State":T11, "Y":dbl})
    n83 = Bundle By Name(cluster=T13 {"connect"=FALSE, "Z_Source"=enum."initialize", "Z_State_heating"=enum."initialization"} ("source"), "connect"=w121, "Z_Source"=w161, "Z_State_heating"=w160) -> (w159:T13)
    n84 = property on="Z_OnSwitch" class="Z_OnSwitch (strict)"() -> ("timer end"=w166:bool)  [unwired: 2 in, 2 out]
    n85 = Bundle By Name(cluster=cluster{"connect":bool, "Z_Source":T9} {"connect"=FALSE, "Z_Source"=enum."initialize"} ("source"), "connect"=w121, "Z_Source"=w161) -> (w151:cluster{"connect":bool, "Z_Source":T9})
    n86 = property on="Z_Hswitch" class="Z_Hswitch (strict)"() -> ("timer end"=w150:bool)  [unwired: 2 in, 2 out]
    n87 = property on="Y_SP" class="Y_SP (strict)"() -> ("timer end"=w127:bool)  [unwired: 2 in, 2 out]
    n88 = Bundle By Name(cluster=cluster{"connect":bool, "Z_Source":T9} {"connect"=FALSE, "Z_Source"=enum."initialize"} ("source"), "connect"=w121, "Z_Source"=w131) -> (w144:cluster{"connect":bool, "Z_Source":T9})
    n89 = property on="Y_Hswitch" class="Z_Hswitch (strict)"() -> ("timer end"=w145:bool)  [unwired: 2 in, 2 out]
    n90 = property on="YQ" class="YQ (strict)"() -> ("timer end"=w141:bool)  [unwired: 2 in, 2 out]
    n91 = case shown="True" w156 {
      tunnel: w132 -> [_ w250]
      frame False {
      }
      frame True {
        n92 = Unbundle By Name(w250) -> ("color"=w251:u32, "visible"=w252:bool)
        n93 = property on="PV" class="Slide (strict)"("Fill Color"=w251) -> ("DigDisps[]"=w255:refnum<vi>[])  [unwired: 2 in, 2 out]
        n94 = Index Array(array=w255, index=0) -> (element=w253:refnum<vi>)
        n95 = property on="Property Node" class="DigNum"(reference=w253, "NumText.BGColor"=w251, "NumText.Visible"=w252) -> ()  [unwired: 1 in, 2 out]
      }
    }
    n96 = local read "name"() -> (w181:string)
    n97 = Not(x=w166) -> (.not. x?=w167:bool)
    n98 = Not(x=w150) -> (.not. x?=w154:bool)
    n99 = Not(x=w127) -> (.not. x?=w125:bool)
    n100 = Not(x=w145) -> (.not. x?=w147:bool)
    n101 = Not(x=w141) -> (.not. x?=w139:bool)
    n102 = call "Is Value Changed.vim"("value"=w159) -> ("changed or first call?"=w162:bool)
    n103 = call "Is Value Changed.vim"("value"=w151) -> ("changed or first call?"=w155:bool)
    n104 = call "Is Value Changed.vim"("value"=w128) -> ("changed or first call?"=w126:bool)
    n105 = call "Is Value Changed.vim"("value"=w144) -> ("changed or first call?"=w146:bool)
    n106 = call "Is Value Changed.vim"("value"=w142) -> ("changed or first call?"=w140:bool)
    n107 = feedback #1() -> (w168:bool)  [unwired: 1 in]
    n108 = feedback-in #1(w167) -> ()
    n109 = feedback #2() -> (w153:bool)  [unwired: 1 in]
    n110 = feedback-in #2(w154) -> ()
    n111 = feedback #3() -> (w124:bool)  [unwired: 1 in]
    n112 = feedback-in #3(w125) -> ()
    n113 = feedback #4() -> (w148:bool)  [unwired: 1 in]
    n114 = feedback-in #4(w147) -> ()
    n115 = feedback #5() -> (w138:bool)  [unwired: 1 in]
    n116 = feedback-in #5(w139) -> ()
    n117 = Unbundle By Name(w134) -> ("Z.ALR  L1"=w164:bool, "Z.ALR  L2"=w163:bool)
    n118 = String Length(string=w181) -> (length=w226:i32)
    n119 = Compound Arithmetic op=OR(w162, w167, w168) -> (w169:bool)
    n120 = Compound Arithmetic op=OR(w155, w154, w153) -> (w152:bool)
    n121 = Compound Arithmetic op=OR(w126, w125, w124) -> (w123:bool)
    n122 = Compound Arithmetic op=OR(w146, w147, w148) -> (w149:bool)
    n123 = Compound Arithmetic op=OR(w140, w139, w138) -> (w137:bool)
    n124 = Index Array(array=string[] ["инициализация", "остановлен", "получен сигнал на пуск", "подан сигнал на включение", "разогрев", "нагреватель включен", "получен сигнал на останов нагревателя (задержка перед отключением)", "снижение нагрузки", "снят сигнал на пуск", "охлаждение", "задержка повторного старта"], index=w173) -> (element=w219:string)
    "Z5 State" <- w219
    n125 = Replace Substring(2:3 ("length (len. of substring)"), 3:15 ("offset (0)"), 4:w181, 5:w231) -> (1:w228:string)  [unwired: 1 out]
    n126 = case shown="True" w137 {
      tunnel: w142 -> [_ w236]
      frame False {
      }
      frame True {
        n127 = property on="YQ" class="YQ (strict)"("State"=w236) -> ()  [unwired: 2 in, 2 out]
      }
    }
    n128 = case shown="True" w152 {
      tunnel: w151 -> [_ w238]
      frame False {
      }
      frame True {
        n129 = property on="Z_Hswitch" class="Z_Hswitch (strict)"("State"=w238) -> ()  [unwired: 2 in, 2 out]
      }
    }
    n130 = case shown="True" w123 {
      tunnel: w128 -> [_ w235]
      frame False {
      }
      frame True {
        n131 = property on="Y_SP" class="Y_SP (strict)"("State"=w235) -> ()  [unwired: 2 in, 2 out]
      }
    }
    n132 = case shown="True" w149 {
      tunnel: w144 -> [_ w237]
      frame False {
      }
      frame True {
        n133 = property on="Y_Hswitch" class="Z_Hswitch (strict)"("State"=w237) -> ()  [unwired: 2 in, 2 out]
      }
    }
    n134 = case shown="True" w169 {
      tunnel: w159 -> [_ w239]
      frame False {
      }
      frame True {
        n135 = property on="Z_OnSwitch" class="Z_OnSwitch (strict)"("State"=w239) -> ()  [unwired: 2 in, 2 out]
      }
    }
    n136 = call "heating_visu_colors.vi"("Z_State"=w160, "Z_Source"=w161) -> ("N ring"=→"Z3 ind":u16)  [unwired: 6 in, 3 out]
    n137 = property on="ALRL1_reset" class="Bool"("Visible"=w164) -> ()  [unwired: 2 in, 2 out]
    n138 = property on="ALRL2_reset" class="Bool"("Visible"=w163) -> ()  [unwired: 2 in, 2 out]
    n139 = Unbundle("Y_SP") -> (w117:dbl)  [unwired: 2 out]
    n140 = Divide(x=w213, y=u32 1000) -> (x/y=→"T stage":dbl)
    n141 = Compound Arithmetic op=ADD(15 ("offset (0)"), w226, 2 ("value")) -> (w224:i32)
    n142 = Replace Substring(2:66 ("value"), 3:w224, 4:w219, 5:w228) -> (1:w223:string)  [unwired: 1 out]
    n143 = Boolean To (0,1)(Boolean="Z_Hswitch") -> (0, 1=w215:i16)
    n144 = Boolean To (0,1)(Boolean="Y_Hswitch") -> (0, 1=w210:i16)
    n145 = Select(t=Z_State."on" ("Z_State"), s="Z_OnSwitch", f=Z_State."stop ready" ("Z_State")) -> (s? t:f=w218:T12)
    n146 = Select(t=Y_state."auto" ("Y_HSetState"), s="Y_Hswitch", f=Y_state."hand" ("Y_HSetState")) -> (s? t:f=w207:T11)
    n147 = Or(x="ALRL1_reset", y="ALRL2_reset") -> (x .or. y?=w203:bool)
    n148 = property on="Z3 ind" class="Ring (strict)"("TipStrip"=w223) -> ()  [unwired: 2 in, 2 out]
    n149 = Bundle By Name(cluster=T16 {"Z_HSw"=0, "Z_HSetState"=0, "Y_HSw"=0, "Y_HSetState"=0, "SP"=0.0, "Y_H"=0.0, "Reset_ALR"=FALSE} ("HT1_in"), "Z_HSw"=w215, "Z_HSetState"=w218, "Y_HSw"=w210, "Y_HSetState"=w207, "SP"=w117, "Y_H"="YQ", "Reset_ALR"=w203) -> (w190:T16)
    n150 = case shown="True" "Write controls" {
      tunnel: w190 -> [_ w266]
      tunnel: w189 -> [w256 w258]
      tunnel: w187 -> [_ w262]
      tunnel: w186 -> [_ w264]
      tunnel: [w256 w260] -> w185
      frame False {
      }
      frame True {
        n151 = Flatten To JSON(anything=w266, error in (no error)=w258) -> (JSON string=w259:string, 11:w257:errorcluster)  [unwired: 1 in]
        n152 = Get Date/Time In Seconds() -> (seconds since 1Jan1904=w265:timestamp)
        n153 = call "Write element.vi"("seconds since 1Jan1904"=w265, "Variant"=w259, "request in"=w264) -> ("request out"=w263:T4)  [unwired: 8 in]
        n154 = Build Array(w263) -> (w261:T4[])
        n155 = call-poly <vilib>:"Multiple Write.vi"("error in (no error)"=w257, "requests"=w261, "OPC UA client refnum in"=w262) -> ("error out"=w260:errorcluster)  [unwired: 5 in, 3 out]
      }
    }
    n156 = control-ref of="This VI"() -> (w198:refnum<vi>)
    "This VI" <- w198
    n157 = disable-structure shown="Disabled" {
      frame Disabled {
      }
      frame Enabled {
      }
    }
    n158 = Wait (ms)(milliseconds to wait=u32 100) -> ()  [unwired: 1 out]
    n159 = global read "Global stop.vi" "Stop"() -> (w201:bool)
    n160 = Compound Arithmetic op=OR(w185, w201, "stop") -> (w184:bool)
    n161 = case shown="True" w184 {
      tunnel: w183 -> [_ w268]
      tunnel: [_ w267] -> w182
      frame False {
      }
      frame True {
        n162 = call <vilib>:"Send Local Message.vi"("message queue in"=w268, "message name"="Exit") -> ("error out"=w267:errorcluster)  [unwired: 11 in, 2 out]
      }
    }
    "Y output" <- "YQ"
  }
  n163 = Merge Errors(w10, w12) -> (w24:errorcluster)
  n164 = disable-structure shown="Disabled" {
    disable-tunnel: w37 -> [w270 _]
    frame Disabled {
      n165 = invoke class="VI" method="FP.Close"(reference=w270) -> ()  [unwired: 2 in, 3 out]
    }
    frame Enabled {
    }
  }
  n166 = call <vilib>:"Delete Monitored Nodes.vi"("error in (no error)"=w24, "node IDs"=w9, "subscription ID in"=w23, "OPC UA client refnum in"=w11) -> ("error out"=w28:errorcluster, "OPC UA client refnum out"=w29:T7)  [unwired: 3 in, 3 out]
  n167 = Build Array(w23) -> (w25:T8[])
  n168 = call <vilib>:"Delete Subscriptions.vi"("error in (no error)"=w28, "subscription IDs"=w25, "OPC UA client refnum in"=w29) -> ("error out"=w26:errorcluster, "OPC UA client refnum out"=w27:T7)  [unwired: 6 in, 1 out]
  n169 = call <vilib>:"Disconnect.vi"("error in (no error)"=w26, "OPC UA client refnum in"=w27) -> ("error out"=w4:errorcluster)  [unwired: 9 in]
  n170 = Merge Errors(w4, w3) -> (→"error out":errorcluster)
